vi "Create Alias and Endpoint List.vi"(10 "Endpoints":string[](array[string]), 11 "Alias Mapping":T1) -> (2 "Endpoint List":string[](array[string]), 3 "Alias List":string[](array[string]))   [LabVIEW 2020, in "Routing and Faulting System Explorer.lvlib"]
uses:
  Routing and Faulting System Explorer.lvlib
  Alias Map by Module.ctl
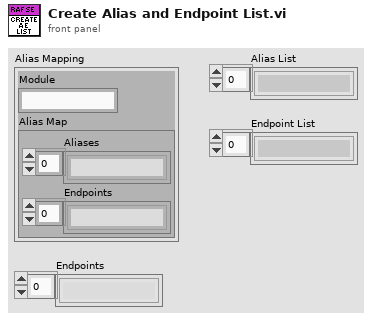
[diagram p1: front panel]
types:
  T1 = typedef "Routing and Faulting System Explorer.lvlib/Alias Map by Module.ctl" = cluster{"Module":string, "Alias Map":cluster{"Aliases":string[], "Endpoints":string[]}}
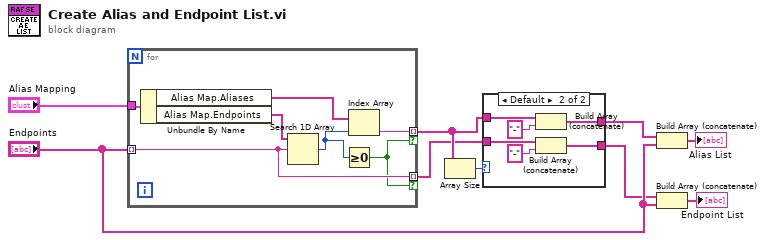
[diagram p0: block diagram]
diagram:
  n1 = for {
    tunnel: "Endpoints" -> [w11] mode=indexing
    tunnel: "Alias Mapping" -> [w16]
    tunnel: [w13] -> w4 mode=indexing if=w10
    tunnel: [w11] -> w3 mode=indexing if=w10
    n2 = Unbundle By Name(w16) -> ("Alias Map.Aliases"=w14:string[], "Alias Map.Endpoints"=w15:string[])
    n3 = Search 1D Array(1D array=w15, element=w11) -> (index of element=w12:i32)  [unwired: 1 in]
    n4 = Greater Or Equal To 0?(x=w12) -> (x >= 0?=w10:bool)
    n5 = Index Array(array=w14, index=w12) -> (element=w13:string)
  }
  n6 = Array Size(array=w4) -> (size(s)=w1:i32)
  n7 = case shown="Default" w1 {
    tunnel: [_ w21] -> w5
    tunnel: w4 -> [_ w20]
    tunnel: w3 -> [_ w18]
    tunnel: [_ w17] -> w6
    frame 0 {
      # "No aliases.\nDon't add\nseparator"
    }
    frame Default {
      n8 = Build Array (concatenate)(w20, "-") -> (w21:string[])
      n9 = Build Array (concatenate)(w18, "-") -> (w17:string[])
    }
  }
  n10 = Build Array (concatenate)(w5, "Endpoints") -> (→"Alias List":string[])
  n11 = Build Array (concatenate)(w6, "Endpoints") -> (→"Endpoint List":string[])
